vi "MakeCenteredEdgeRect.vi"(8 "错误输入":errorcluster, 9 "edge":T1 caption="边缘", 11 "rect":T2 caption="矩形") -> (0 "错误输出":errorcluster, 3 "edge rect":T2 caption="边缘矩形")   [LabVIEW 2012, in "Picture Box Tools.lvlib" / "Rect Tools.lvlib"]
uses:
  Rect Tools.lvlib
  EdgeEnum.ctl
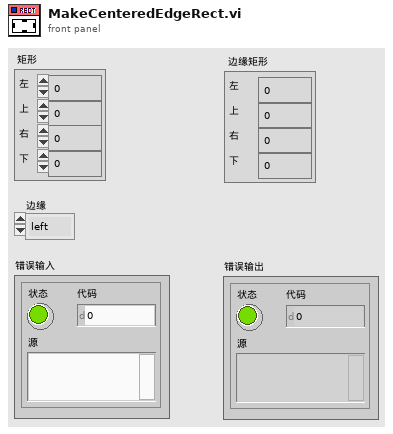
[diagram p1: front panel]
types:
  T1 = typedef "Picture Box Tools.lvlib/Rect Tools.lvlib/EdgeEnum.ctl" = enum16{"left", "top", "right", "bottom"}
  T2 = cluster{"left":i16, "top":i16, "right":i16, "bottom":i16}
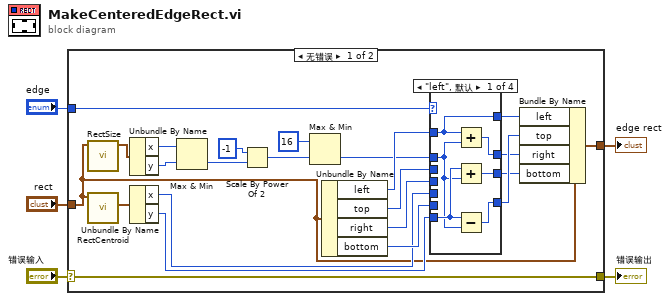
[diagram p0: block diagram]
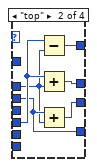
[diagram p2: hidden frame]
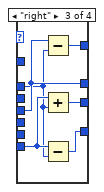
[diagram p3: hidden frame]
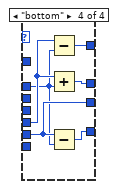
[diagram p4: hidden frame]
diagram:
  n1 = case shown="无错误" "错误输入" {
    selector: "错误输入" -> [w9 w53]
    tunnel: [w9 w53] -> w4
    tunnel: "rect" -> [w8 _]
    tunnel: [w7 _] -> w2
    tunnel: "edge" -> [w6 _]
    frame No Error {
      n2 = call "RectSize.vi"("rect"=w8) -> ("point"=w17:cluster{"x":i16, "y":i16})  [unwired: 7 in, 3 out]
      n3 = call "RectCentroid.vi"("Rect In"=w8) -> ("point"=w20:cluster{"x":i16, "y":i16})  [unwired: 8 in, 2 out]
      n4 = Unbundle By Name(w17) -> ("x"=w16:i16, "y"=w15:i16)
      n5 = Unbundle By Name(w20) -> ("x"=w19:i16, "y"=w18:i16)
      n6 = Max & Min(x=w16, y=w15) -> (min(x,y)=w14:i16)  [unwired: 1 out]
      n7 = Scale By Power Of 2(n=-1, x=w14) -> (x*2^n=w12:i16)
      n8 = Max & Min(x=i16 16, y=w12) -> (min(x,y)=w10:i16)  [unwired: 1 out]
      n9 = Unbundle By Name(w8) -> ("left"=w23:i16, "top"=w26:i16, "right"=w21:i16, "bottom"=w25:i16)
      n10 = case shown="\"left\", 默认" w6 {
        tunnel: [w30 w36 w42 w51] -> w28
        tunnel: [w31 w40 w43 w52] -> w27
        tunnel: w26 -> [_ w36 _ _]
        tunnel: w25 -> [_ _ _ w52]
        tunnel: [w33 w37 w45 w49] -> w24
        tunnel: w23 -> [w33 _ _ _]
        tunnel: [w34 w38 w44 w48] -> w22
        tunnel: w21 -> [_ _ w44 _]
        tunnel: w19 -> [_ w39 _ w50]
        tunnel: w18 -> [w32 _ w46 _]
        tunnel: w10 -> [w29 w35 w41 w47]
        frame "left", Default {
          n11 = Add(x=w33, y=w29) -> (x+y=w34:i16)
          n12 = Add(x=w32, y=w29) -> (x+y=w31:i16)
          n13 = Subtract(x=w32, y=w29) -> (x-y=w30:i16)
        }
        frame "top" {
          n14 = Subtract(x=w39, y=w35) -> (x-y=w37:i16)
          n15 = Add(x=w39, y=w35) -> (x+y=w38:i16)
          n16 = Add(x=w36, y=w35) -> (x+y=w40:i16)
        }
        frame "right" {
          n17 = Subtract(x=w44, y=w41) -> (x-y=w45:i16)
          n18 = Add(x=w46, y=w41) -> (x+y=w43:i16)
          n19 = Subtract(x=w46, y=w41) -> (x-y=w42:i16)
        }
        frame "bottom" {
          n20 = Subtract(x=w50, y=w47) -> (x-y=w49:i16)
          n21 = Add(x=w50, y=w47) -> (x+y=w48:i16)
          n22 = Subtract(x=w52, y=w47) -> (x-y=w51:i16)
        }
      }
      n23 = Bundle By Name(cluster=w8, "left"=w24, "top"=w28, "right"=w22, "bottom"=w27) -> (w7:T2)
    }
    frame Error {
    }
  }
  "错误输出" <- w4
  "edge rect" <- w2
